vi "V_GLOB2.vi"() -> ()   [LabVIEW 2017]
panel:
  out "POSICIONA":dbl
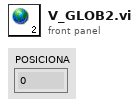
[diagram p1: front panel]
diagram:
